vi "global variable-賭金金額.vi"() -> ()   [LabVIEW 2014]
panel:
  in  "賭金金額":i32
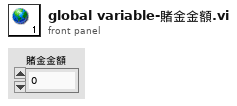
[diagram p1: front panel]
diagram:
